vi "GetTracepointsDirectory.vi"(8 "error in (no error)":errorcluster) -> (0 "error out":errorcluster, 3 "application directory":path)   [LabVIEW 2017]
doc: "Returns the path of the directory where the device stores configuration JSON files from the server."
uses:
  <vilib>/addons/PointValueMap/subVIs/Point_Read_variant.vi
  <vilib>/addons/PointValueMap/subVIs/Point_Write_variant.vi
  <vilib>/addons/PointValueMap/PointValueMap.lvlib
  <vilib>/addons/InsightCM/Utilities/GlobalConfiguration/GlobalConfiguration.lvlib
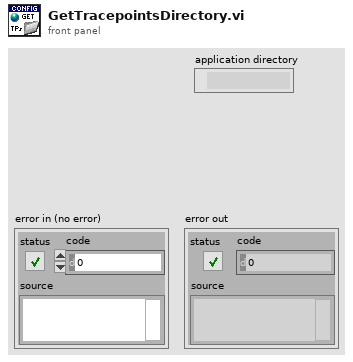
[diagram p1: front panel]
types:
  T1 = typedef "PointValueMap.lvlib/PointMap.ctl" = refnum<data-value>
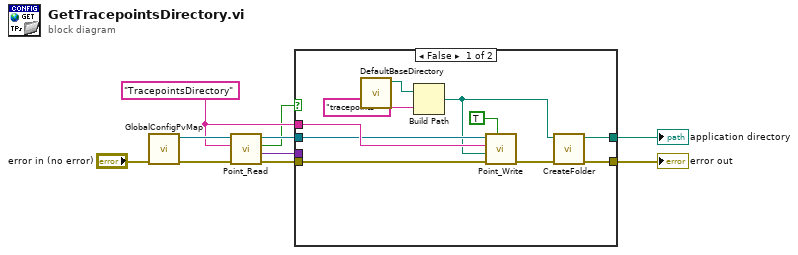
[diagram p0: block diagram]
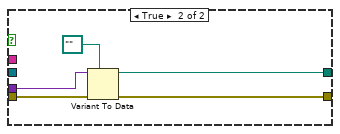
[diagram p2: hidden frame]
diagram:
  w6 = "TracepointsDirectory" ("Name")
  n1 = call <vilib>:"GlobalConfigPvMap.vi"("error in (no error)"="error in (no error)") -> ("error out"=w4:errorcluster, "global configuration map"=w8:T1)  [unwired: 9 in]
  n2 = call-poly <vilib>:"Point_Read.vi"("Error In"=w4, "Tag"=w6, "Map"=w8) -> ("Error Out"=w3:errorcluster, "Value"=w2:variant, "Found?"=w1:bool, "Map Out"=w5:T1)  [unwired: 3 in, 2 out]
  n3 = case shown="False" w1 {
    tunnel: [w11 w25] -> w10
    tunnel: [w12 w24] -> w7
    tunnel: w6 -> [w18 _]
    tunnel: w5 -> [w17 _]
    tunnel: w3 -> [w15 w22]
    tunnel: w2 -> [_ w21]
    frame False {
      n4 = call <vilib>:"DefaultBaseDirectory.vi"() -> ("base directory"=w20:path)  [unwired: 11 in]
      n5 = Build Path(base path=w20, name or relative path="tracepoints") -> (appended path=w13:path)
      n6 = call-poly <vilib>:"Point_Write.vi"("Auto Create?"=TRUE, "Error In"=w15, "Value"=w13, "Tag"=w18, "Map"=w17) -> ("Error Out"=w14:errorcluster)  [unwired: 5 in, 1 out]
      n7 = call <vilib>:"CreateFolder.vi"("error in (no error)"=w14, "folder"=w13) -> ("error out"=w11:errorcluster, "folder out"=w12:path)  [unwired: 8 in]
    }
    frame True {
      n8 = Variant To Data(error in=w22, type=path "", Variant=w21) -> (data=w24:path, error out=w25:errorcluster)
    }
  }
  "error out" <- w10
  "application directory" <- w7
